vi "Set Motor Velocity.vi"(0 "Acceleration ramp constant":dbl(slide)=10.303030303030303 scale=0.0..20.0, 1 "Accelerate?":bool=TRUE, 4 "Back motor speed rev/s":dbl, 6 "Motor Controller PID Gains Right":T1={"P Gain"=0.2, "I Gain"=0.0, "D Gain"=0.0}, 7 "Motor Controller PID Gains Left":T1={"P Gain"=0.2, "I Gain"=0.0, "D Gain"=0.0}, 8 "Disable motors":bool, 9 "dt":dbl=0.02, 10 "Right motor speed rev/s":dbl, 11 "Left motor speed rev/s":dbl) -> ()   [LabVIEW 2016]
uses:
  <vilib>/addons/control/pid/pid.llb/PID (DBL).vi
  <vilib>/addons/control/pid/NI_PID_pid.lvlib
panel:
  out "Encoder Values":cluster{"Left  Value":i32, "Right Value":i32}(graph)
  out "Waveform Chart":cluster{"Left  Value":dbl, "Right Value":dbl}(graph)
  in  "Bypass PID":bool
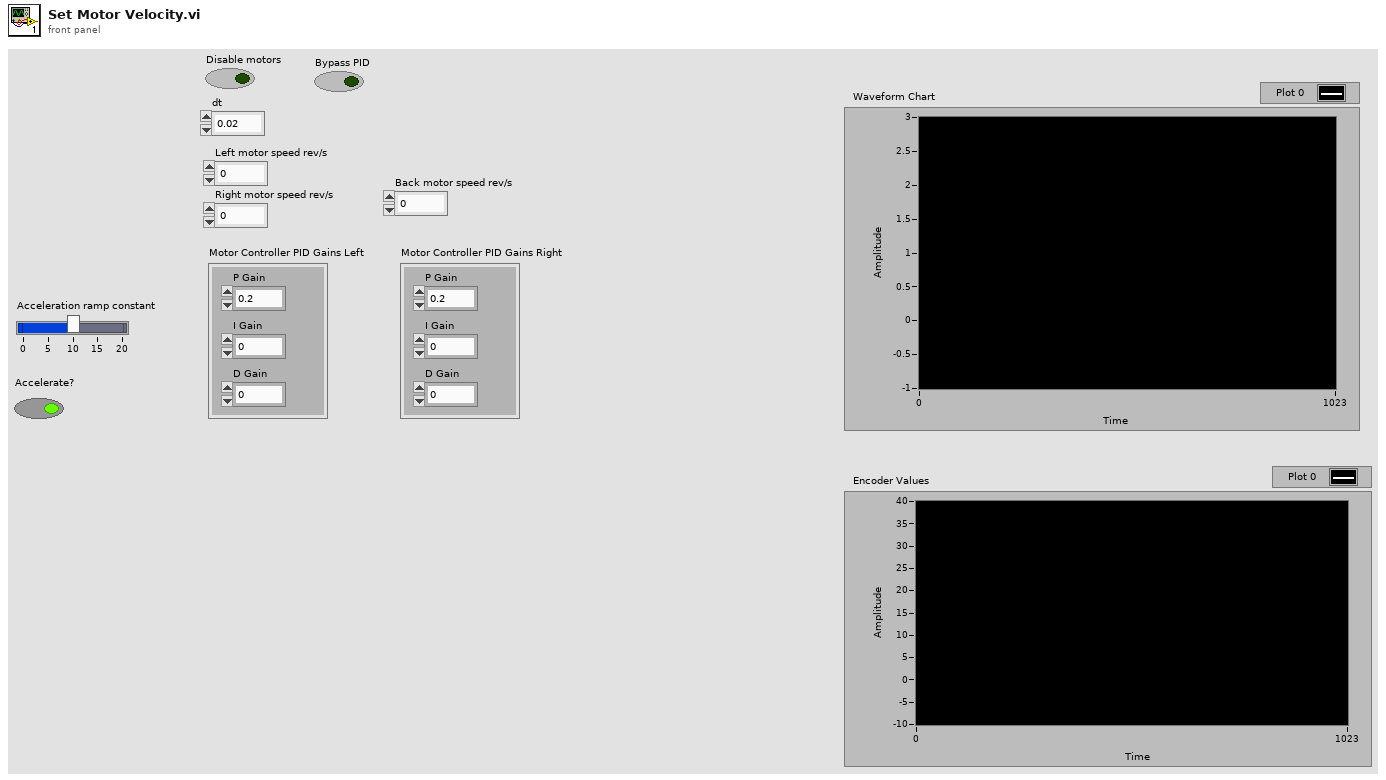
[diagram p1: front panel]
types:
  T1 = cluster{"P Gain":dbl, "I Gain":dbl, "D Gain":dbl}
  T2 = cluster{"Left motor speed rev/s":dbl, "Right motor speed rev/s":dbl, "Back motor speed rev/s":dbl}
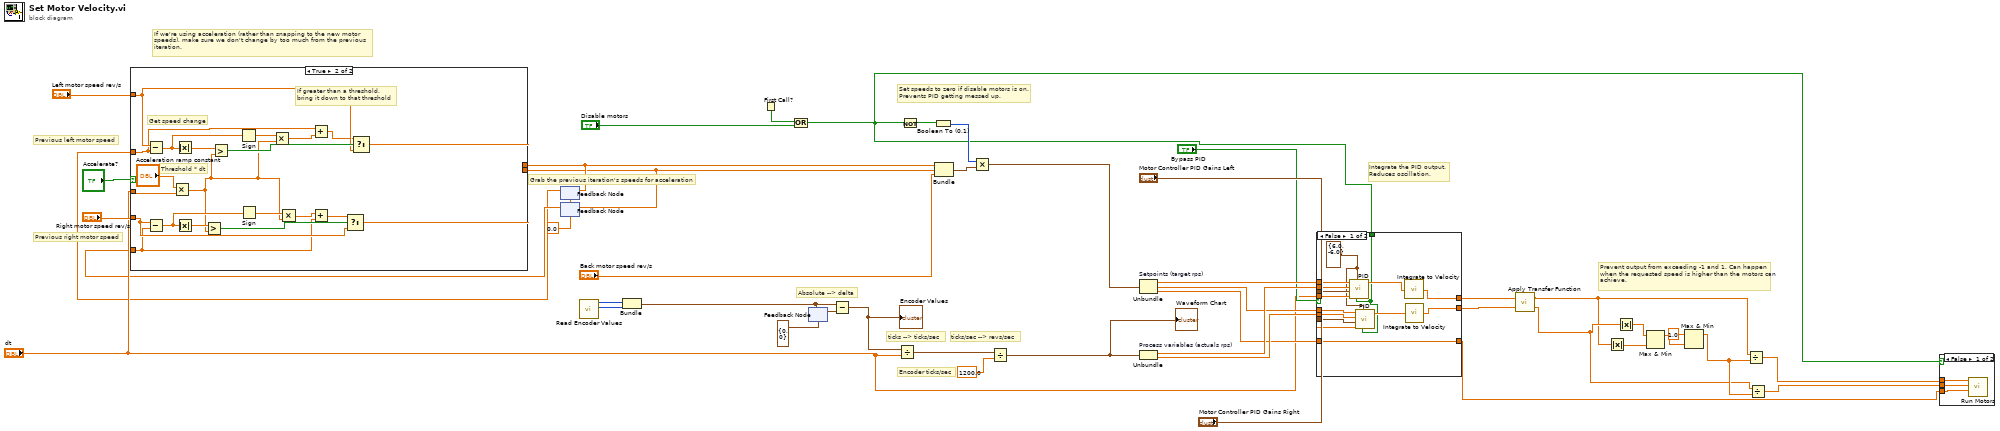
[diagram p0: block diagram]
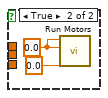
[diagram p4: hidden frame]
diagram:
  w7 = 0.0
  # "Previous right motor speed"
  # "Previous left motor speed"
  # "Grab the previous iteration's speeds for acceleration"
  # "If we're using acceleration (rather than snapping to the new motor\nspeeds), make sure we don't change by too much from the previous\niteration."
  # "Integrate the PID output.\nReduces oscillation."
  # "ticks --> ticks/sec"
  # "Set speeds to zero if disable motors is on.\nPrevents PID getting messed up."
  # "Prevent output from exceeding -1 and 1. Can happen when the requested speed is higher than the motors can achieve."
  # "Encoder ticks/sec"
  # "ticks/sec --> revs/sec"
  # "Absolute --> delta"
  n1 = feedback #1(w7) -> (w2:dbl)
  n2 = feedback #2(w7) -> (w3:dbl)
  n3 = case shown="True" "Accelerate?" {
    tunnel: [w47 w59] -> w5
    tunnel: [w48 w65] -> w6
    tunnel: "Left motor speed rev/s" -> [w48 w64]
    tunnel: "Right motor speed rev/s" -> [w47 w58]
    tunnel: w2 -> [_ w53]
    tunnel: w3 -> [_ w50]
    tunnel: "dt" -> [_ w56]
    frame False {
    }
    frame True {
      # "Threshold * dt"
      # "If greater than a threshold,\nbring it down to that threshold"
      # "Get speed change"
      n4 = Subtract(x=w64, y=w53) -> (x-y=w67:dbl)
      n5 = Subtract(x=w58, y=w50) -> (x-y=w60:dbl)
      n6 = Multiply(x="Acceleration ramp constant", y=w56) -> (x*y=w55:dbl)
      n7 = Absolute Value(x=w67) -> (abs(x)=w69:dbl)
      n8 = Absolute Value(x=w60) -> (abs(x)=w63:dbl)
      n9 = Greater?(x=w63, y=w55) -> (0:w62:bool)
      n10 = Greater?(x=w69, y=w55) -> (0:w68:bool)
      n11 = Sign(1:w67) -> (0:w66:dbl)
      n12 = Sign(1:w60) -> (0:w61:dbl)
      n13 = Multiply(x=w66, y=w55) -> (x*y=w52:dbl)
      n14 = Multiply(x=w61, y=w55) -> (x*y=w51:dbl)
      n15 = Add(x=w53, y=w52) -> (x+y=w54:dbl)
      n16 = Add(x=w51, y=w50) -> (x+y=w49:dbl)
      n17 = Select(t=w49, s=w62, f=w58) -> (s? t:f=w59:dbl)
      n18 = Select(t=w54, s=w68, f=w64) -> (s? t:f=w65:dbl)
    }
  }
  n19 = feedback-in #1(w6) -> ()
  n20 = feedback-in #2(w5) -> ()
  n21 = call "Read Encoder Values.vi"() -> ("Right Value"=w31:i32, "Left  Value"=w32:i32)  [unwired: 10 in]
  n22 = Bundle("Left  Value"=w32, "Right Value"=w31) -> (w42:cluster{"Left  Value":i32, "Right Value":i32})  [unwired: 1 in]
  n23 = First Call?() -> (First Call?: T/F=w45:bool)
  n24 = Or(x=w45, y="Disable motors") -> (x .or. y?=w1:bool)
  n25 = feedback #3(cluster{"Left  Value":i32, "Right Value":i32} {"Left  Value"=0, "Right Value"=0}) -> (w41:cluster{"Left  Value":i32, "Right Value":i32})
  n26 = feedback-in #3(w42) -> ()
  n27 = Subtract(x=w42, y=w41) -> (x-y=w11:cluster{"Left  Value":i32, "Right Value":i32})
  "Encoder Values" <- w11
  n28 = Divide(x=w11, y="dt") -> (x/y=w46:cluster{"Left  Value":dbl, "Right Value":dbl})
  n29 = Not(x=w1) -> (.not. x?=w30:bool)
  n30 = Boolean To (0,1)(Boolean=w30) -> (0, 1=w25:i16)
  n31 = Bundle("Left motor speed rev/s"=w6, "Right motor speed rev/s"=w5, "Back motor speed rev/s"="Back motor speed rev/s") -> (w24:T2)  [unwired: 1 in]
  n32 = Multiply(x=w25, y=w24) -> (x*y=w23:T2)
  n33 = Divide(x=w46, y=1200.0 ("Left  Value")) -> (x/y=w19:cluster{"Left  Value":dbl, "Right Value":dbl})
  "Waveform Chart" <- w19
  n34 = Unbundle "Setpoints (target rps)"(w23) -> ("Left motor speed rev/s"=w28:dbl, "Right motor speed rev/s"=w27:dbl, "Back motor speed rev/s"=w13:dbl)
  n35 = Unbundle "Process variables (actuals rps)"(w19) -> ("Left  Value"=w29:dbl, "Right Value"=w26:dbl)
  n36 = case shown="False" "Bypass PID" {
    tunnel: w29 -> [w83 _]
    tunnel: w28 -> [w82 w86]
    tunnel: w27 -> [w81 w85]
    tunnel: w26 -> [w80 _]
    tunnel: "dt" -> [w79 _]
    tunnel: [w75 w86] -> w18
    tunnel: [w73 w85] -> w17
    tunnel: "Motor Controller PID Gains Left" -> [w78 _]
    tunnel: "Motor Controller PID Gains Right" -> [w77 _]
    tunnel: w13 -> [w72 w84]
    tunnel: [w72 w84] -> w12
    tunnel: w1 -> [w71 _]
    frame False {
      w70 = cluster{"output high":dbl, "output low":dbl} {"output high"=6.0, "output low"=-6.0} ("output range")
      n37 = call-poly <vilib>:"PID.vi"("reinitialize? (F)"=w71, "output range"=w70, "dt (s)"=w79, "PID gains"=w78, "process variable"=w83, "setpoint"=w82) -> ("output"=w76:dbl)  [unwired: 4 in, 1 out]
      n38 = call-poly <vilib>:"PID.vi"("reinitialize? (F)"=w71, "output range"=w70, "dt (s)"=w79, "PID gains"=w77, "process variable"=w80, "setpoint"=w81) -> ("output"=w74:dbl)  [unwired: 4 in, 1 out]
      n39 = call "Integrate to Velocity.vi"("x"=w76) -> ("Output"=w75:dbl)
      n40 = call "Integrate to Velocity.vi"("x"=w74) -> ("Output"=w73:dbl)
    }
    frame True {
    }
  }
  n41 = call "Apply Transfer Function.vi"("Right Motor"=w17, "Left Motor"=w18) -> ("Right Motor Voltage"=w16:dbl, "Left Motor Voltage"=w15:dbl)
  n42 = Absolute Value(x=w15) -> (abs(x)=w38:dbl)
  n43 = Absolute Value(x=w16) -> (abs(x)=w39:dbl)
  n44 = Max & Min(x=w39, y=w38) -> (max(x,y)=w37:dbl)  [unwired: 1 out]
  n45 = Max & Min(x=1.0, y=w37) -> (max(x,y)=w35:dbl)  [unwired: 1 out]
  n46 = Divide(x=w15, y=w35) -> (x/y=w34:dbl)
  n47 = Divide(x=w16, y=w35) -> (x/y=w33:dbl)
  n48 = case shown="False" w1 {
    tunnel: w34 -> [w89 _]
    tunnel: w33 -> [w88 _]
    tunnel: w12 -> [w87 _]
    frame False {
      n49 = call "Run Motors.vi"("Back motor (-1..1)"=w87, "Right motor side (-1..1)"=w88, "Left motor speed (-1..1)"=w89) -> ()  [unwired: 9 in]
    }
    frame True {
      w91 = 0.0 ("Left motor speed (-1..1)")
      n50 = call "Run Motors.vi"("Back motor (-1..1)"=0.0, "Right motor side (-1..1)"=w91, "Left motor speed (-1..1)"=w91) -> ()  [unwired: 9 in]
    }
  }
